vi "Load Sub Panel.vi"(8 "error in (no error)":errorcluster, 10 "sub panel ref":refnum<vi>, 11 "Logger in":refnum<class "Logger.lvclass">) -> (0 "error out":errorcluster, 3 "Logger out":refnum<class "Logger.lvclass">)   [LabVIEW 2020, in "Logger.lvlib" / "Logger.lvclass"]
uses:
  Logger.lvclass
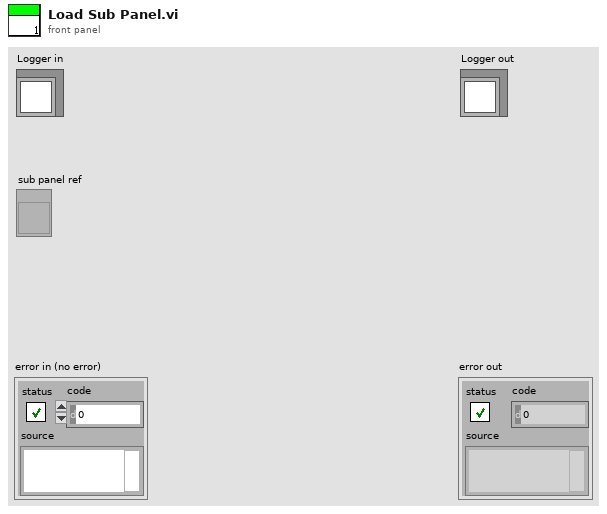
[diagram p1: front panel]
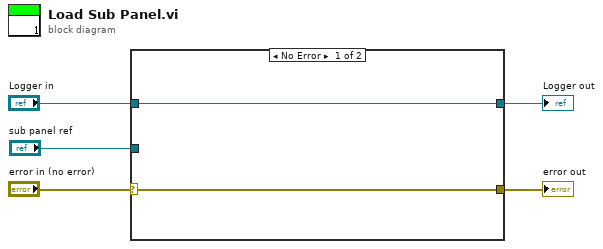
[diagram p0: block diagram]
diagram:
  n1 = case shown="No Error" "error in (no error)" {
    selector: "error in (no error)" -> [w6 w9]
    tunnel: [w6 w9] -> w4
    tunnel: [w7 w8] -> w2
    tunnel: "Logger in" -> [w7 w8]
    tunnel: "sub panel ref" -> [_ _]
    frame No Error {
    }
    frame Error {
    }
  }
  "error out" <- w4
  "Logger out" <- w2
